vi "LEP_RV_SetDebugSymbol.vi"(8 "error in":errorcluster, 11 "debug":bool=TRUE) -> (0 "error out":errorcluster)   [LabVIEW 2011]
uses:
  <vilib>/Platform/EmbProject/Plugins/utilities/LEP_Utilities_GetSetProjectData_String.vi
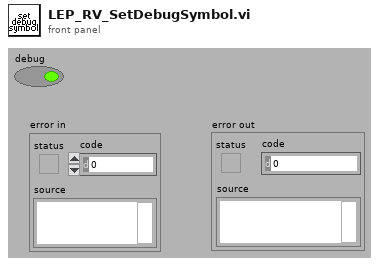
[diagram p1: front panel]
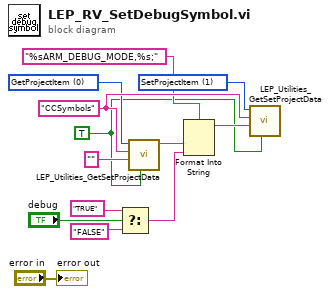
[diagram p0: block diagram]
diagram:
  w8 = u16 0 items=["GetProjectItem", "SetProjectItem"] ("Command")
  w13 = u16 1 items=["GetProjectItem", "SetProjectItem"] ("Command")
  w2 = TRUE ("access target data (F)")
  w9 = "CCSymbols" ("Name")
  n1 = Select(t="TRUE" ("Name"), s="debug", f="FALSE" ("Name")) -> (s? t:f=w4:string)
  n2 = call-poly <vilib>:"LEP_Utilities_GetSetProjectData.vi"("access target data (F)"=w2, "data in"="" ("Name"), "ItemName"=w9, "Command"=w8) -> ("data out"=w5:string)  [unwired: 1 in, 6 out]
  n3 = Format Into String(format string="%sARM_DEBUG_MODE,%s;", w5, w4) -> (resulting string=w3:string)  [unwired: 2 in, 1 out]
  n4 = call-poly <vilib>:"LEP_Utilities_GetSetProjectData.vi"("access target data (F)"=w2, "data in"=w3, "ItemName"=w9, "Command"=w13) -> ()  [unwired: 1 in, 7 out]
  "error out" <- "error in"
